vi "Up_CreatePattern.vi"(10 "Enum_ROI_Select":T3, 11 "ROI":T2) -> (3 "Image Out":T1(plugin-control))   [LabVIEW 2019]
uses:
  Ctrl/UpROIName.ctl
  Ctrl/UpGrayImg.ctl
  Ctrl/UpColorImg.ctl
  LLB/Commonly VI/Main Glb.vi
  LLB/Commonly VI/Load Glb.vi
  <vilib>/vision/NI_Vision_Development_Module.lvlib
  LLB/Commonly VI.lvlib
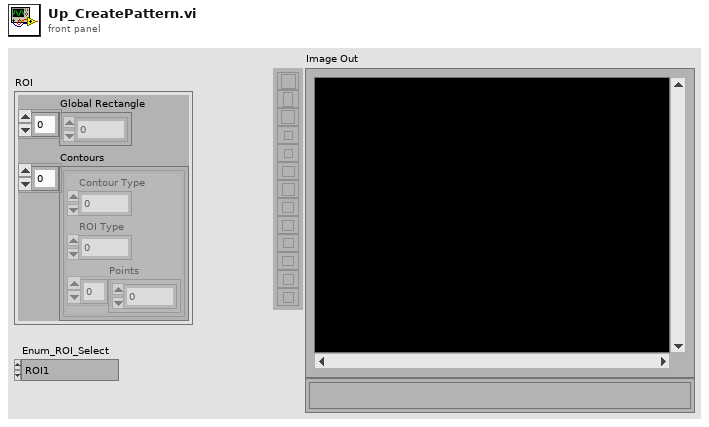
[diagram p1: front panel]
types:
  T1 = typedef "IMAQ Image.ctl" = refnum<image>
  T2 = cluster{"Global Rectangle":i32[], "Contours":cluster{"Contour Type":u32, "ROI Type":u32, "Points":i32[]}[]}
  T3 = typedef "UpROIName.ctl" = enum16{"ROI1", "ROI2", "ROI3"}
  T4 = typedef "UpColorImg.ctl" = enum16{"CUpCam", "CUpSource", "CUpShow", "CUpToProcess1", "CUpToProcess2", "CUpForMatch", "CUpForCheckNumbers", "CupPreProcess"}
  T5 = typedef "UpGrayImg.ctl" = enum16{"CUpGray", "CUpProce1", "CUpProce2", "UpPattern1", "UpPattern2", "UpCalibImg", "UpPreProcess"}
  T6 = typedef "Image Type" = u32
  T7 = typedef "IMAQ Rectangle" = cluster{"Left":i32, "Top":i32, "Right":i32, "Bottom":i32, "Rotation":dbl}
  T8 = typedef "ROI Descriptor" = cluster{"Global Rectangle":i32[], "Contours":cluster{"ID":enum32{"External", "Internal"}, "Type":u32, "Coordinates":i32[]}[]}
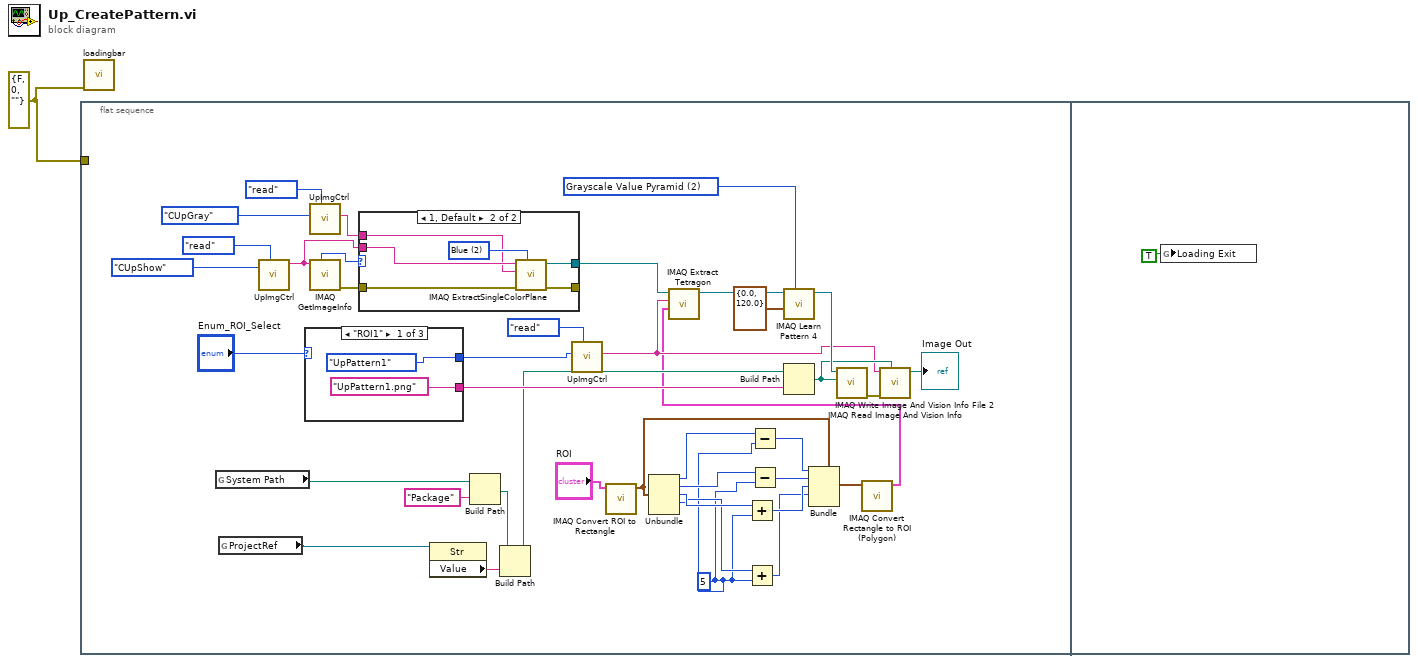
[diagram p0: block diagram]
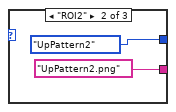
[diagram p2: hidden frame]
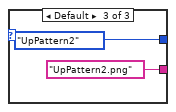
[diagram p3: hidden frame]
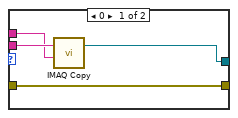
[diagram p4: hidden frame]
diagram:
  w1 = errorcluster {"status"=FALSE, "code"=0, "source"=""} ("error constant")
  n1 = flat-sequence {
    tunnel: w1 -> [_]
    frame #0 {
      w11 = 5 ("y")
      w29 = 2 items=["All", "Low Discrepancy Sampling", "Grayscale Value Pyramid", "Gradients Pyramid"] ("Algorithm")
      n2 = global read "Main Glb.vi" "System Path"() -> (w3:path)
      n3 = global read "Main Glb.vi" "ProjectRef"() -> (w2:refnum<vi>)
      n4 = call "UpImgCtrl.vi"("Action"=enum16{"Initial", "read", "release"}."read", "ColorImg 2"=UpColorImg."CUpShow") -> ("ColorImg"=w22:string)  [unwired: 7 in, 2 out]
      n5 = case shown="\"ROI1\"" "Enum_ROI_Select" {
        tunnel: [UpGrayImg."UpPattern1" ("GrayImg 2") UpGrayImg."UpPattern2" ("GrayImg 2") UpGrayImg."UpPattern2" ("GrayImg 2")] -> w40
        tunnel: ["UpPattern1.png" "UpPattern2.png" "UpPattern2.png"] -> w27
        frame "ROI1" {
        }
        frame "ROI2" {
        }
        frame Default {
        }
      }
      n6 = call "UpImgCtrl.vi"("Action"=enum16{"Initial", "read", "release"}."read", "GrayImg 2"=UpGrayImg."CUpGray" ("GrayImg")) -> ("GrayImg"=w37:string)  [unwired: 7 in, 2 out]
      n7 = call "IMAQ GetImageInfo"("Image"=w22) -> ("error out"=w34:errorcluster, "Image Type"=w33:T6)  [unwired: 3 in, 6 out]
      n8 = case shown="1, Default" w33 {
        tunnel: [w51 w57] -> _
        tunnel: [w48 w56] -> w38
        tunnel: w34 -> [w51 w55]
        tunnel: w22 -> [w50 w54]
        tunnel: w37 -> [w49 w52]
        frame 0 {
          n9 = call "IMAQ Copy"("Image Dst"=w49, "Image Src"=w50) -> ("Image Dst Out"=w48:T1)  [unwired: 4 in, 1 out]
        }
        frame 1, Default {
          w53 = 2 items=["Red", "Green", "Blue", "Hue", "Saturation", "Luminance", "Value", "Intensity"] ("Color Plane")
          n10 = call "IMAQ ExtractSingleColorPlane"("Color Plane"=w53, "error in (no error)"=w55, "Image Dst"=w52, "Image Src"=w54) -> ("error out"=w57:errorcluster, "Image Dst Out"=w56:T1)  [unwired: 6 out]
        }
      }
      n11 = property class="Str"(reference=w2) -> ("Value"=w31:string)  [unwired: 1 in, 2 out]
      n12 = Build Path(base path=w3, name or relative path="Package") -> (appended path=w19:path)
      n13 = Build Path(base path=w19, name or relative path=w31) -> (appended path=w21:path)
      n14 = call "UpImgCtrl.vi"("Action"=enum16{"Initial", "read", "release"}."read", "GrayImg 2"=w40) -> ("GrayImg"=w24:string)  [unwired: 7 in, 2 out]
      n15 = call "IMAQ Convert ROI to Rectangle"("ROI Descriptor"="ROI") -> ("Rectangle"=w10:T7)  [unwired: 8 in, 1 out]
      n16 = Unbundle(w10) -> ("Left"=w15:i32, "Top"=w14:i32, "Right"=w13:i32, "Bottom"=w12:i32)  [unwired: 1 out]
      n17 = Add(x=w13, y=w11) -> (x+y=w7:i32)
      n18 = Add(x=w12, y=w11) -> (x+y=w6:i32)
      n19 = Subtract(x=w15, y=w11) -> (x-y=w9:i32)
      n20 = Subtract(x=w14, y=w11) -> (x-y=w8:i32)
      n21 = Build Path(base path=w21, name or relative path=w27) -> (appended path=w26:path)
      n22 = Bundle(cluster=w10, "Left"=w9, "Top"=w8, "Right"=w7, "Bottom"=w6) -> (w5:T7)  [unwired: 1 in]
      n23 = call "IMAQ Convert Rectangle to ROI (Polygon)"("Rectangle"=w5) -> ("ROI Descriptor"=w4:T8)  [unwired: 7 in, 2 out]
      n24 = call-poly "IMAQ Extract Tetragon"("ROI Descriptor"=w4, "Image Dst"=w24, "Image Src"=w38) -> ("Image Dst Out"=w30:T1)  [unwired: 7 in, 1 out]
      n25 = call "IMAQ Learn Pattern 4"("Algorithm"=w29, "Angle Range"=cluster{"Start Angle":sgl, "End Angle":sgl} {"Start Angle"=0.0, "End Angle"=120.0}, "Image"=w30) -> ("Template Image Out"=w28:T1)  [unwired: 6 in, 2 out]
      n26 = call "IMAQ Write Image And Vision Info File 2"("File Path"=w26, "Image"=w28) -> ("error out"=w25:errorcluster)  [unwired: 8 in, 1 out]
      n27 = call "IMAQ Read Image And Vision Info"("File Path"=w26, "error in (no error)"=w25, "Image"=w24) -> ("Image Out"=→"Image Out":T1)  [unwired: 6 in, 2 out]
    }
    frame #1 {
      n28 = global write "Load Glb.vi" "Loading Exit"(TRUE ("LoadingExit")) -> ()
    }
  }
  n29 = call "loadingbar.vi"("error in"=w1) -> ()  [unwired: 10 in, 1 out]
